vi "HP 3458 multiple digitizer.vi"() -> ()   [LabVIEW 2019]
panel:
  in  "VISA session":refnum<visa-resource-name>
  in  "?":dbl[](array[numeric]) format="%.2f"
  in  "Time Spacing":dbl=0.00025 format="%.3e"
  in  "# Points":u32=4000
  out "?":cluster{dbl, "Time Spacing":dbl, dbl[]}(graph)
  out "Measurement":dbl[](array[numeric]) format="%.5e"
  in  "number of calls":u32
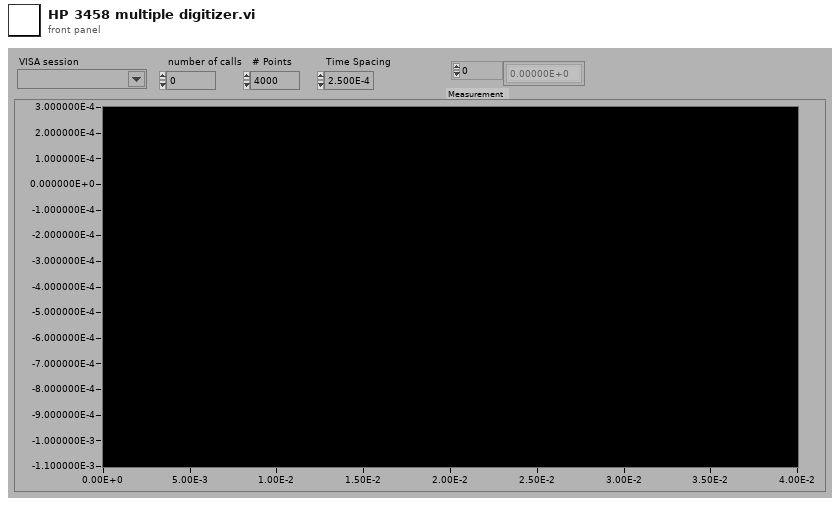
[diagram p1: front panel]
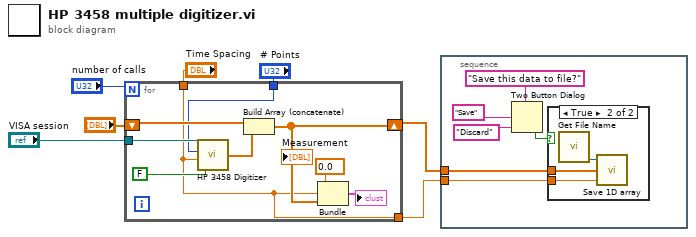
[diagram p0: block diagram]
diagram:
  n1 = for {
    N: "number of calls" -> [_]
    shift-right: [w14] -> w2
    shift-left: "?" -> [w15]
    tunnel: "Time Spacing" -> [w9]
    tunnel: "VISA session" -> [w12]
    tunnel: "# Points" -> [w11]
    tunnel: [w9] -> w1
    n2 = call "HP 3458 Digitizer.vi"("Ask Save Data"=FALSE, "Time Spacing"=w9, "# Points"=w11, "VISA session"=w12) -> ("Measurement"=w16:dbl[])
    n3 = Build Array (concatenate)(w15, w16) -> (w14:dbl[])
    "Measurement" <- w14
    n4 = Bundle(0.0, "Time Spacing"=w9, w14) -> (→"?":cluster{dbl, "Time Spacing":dbl, dbl[]})  [unwired: 1 in]
  }
  n5 = stacked-sequence {
    tunnel: w2 -> [w18]
    tunnel: w1 -> [w17]
    frame #0 {
      n6 = Two Button Dialog(message="Save this data to file?", 1:"Discard", 2:"Save") -> (T button?=w22:bool)
      n7 = case shown="True" w22 {
        tunnel: w18 -> [_ w24]
        tunnel: w17 -> [_ w23]
        frame False {
        }
        frame True {
          n8 = call "Get File Name.vi"() -> (w25:path)
          n9 = call "Save 1D array.vi"("ÆT"=w23, "Data"=w24, "File Path"=w25) -> ()
        }
      }
    }
  }
